vi "Str2HexStrU8.vi"(11 "データ":string) -> (1 "符号なしバイト配列":u8[](array[numeric]) format="%02x", 3 "文字列出力":string)   [LabVIEW 2015]
uses:
  <vilib>/Utility/error.llb/whitespace.ctl
panel:
  # "C0 FF 01 ･･･"
  # "U8を文字列扱い\nしたもの"
  # "16進、区切りスペースの文字列"
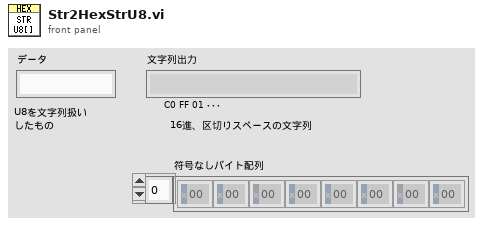
[diagram p1: front panel]
types:
  T1 = typedef "whitespace.ctl" = u16
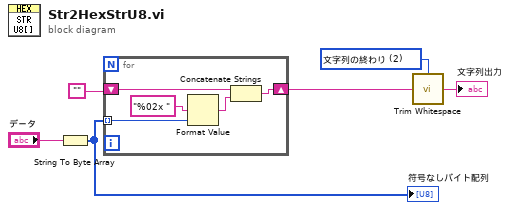
[diagram p0: block diagram]
diagram:
  w3 = T1 2 items=["両方", "文字列の先頭", "文字列の終わり"] ("location (both)")
  n1 = String To Byte Array(string="データ") -> (unsigned byte array=w2:u8[])
  "符号なしバイト配列" <- w2
  n2 = for {
    tunnel: w2 -> [w11] mode=indexing
    shift-right: [w9] -> w5
    shift-left: "" -> [w8]
    n3 = Format Value(format string="%02x ", value (0)=w11) -> (output string=w7:string)  [unwired: 1 in]
    n4 = Concatenate Strings(w8, w7) -> (w9:string)
  }
  n5 = call <vilib>:"Trim Whitespace.vi"("string"=w5, "location (both)"=w3) -> ("trimmed string"=→"文字列出力":string)
